vi "Reports.vi"(8 "Reports":T1(array[cluster]), 9 "Path In":path) -> ()   [LabVIEW 2018]
panel:
  out "Failed":bool
  out "Numeric 2":dbl
  out "String":string="C:\\LabVIEW_Data\\Default.txt"
  out "Numeric":dbl
  out "Output":string
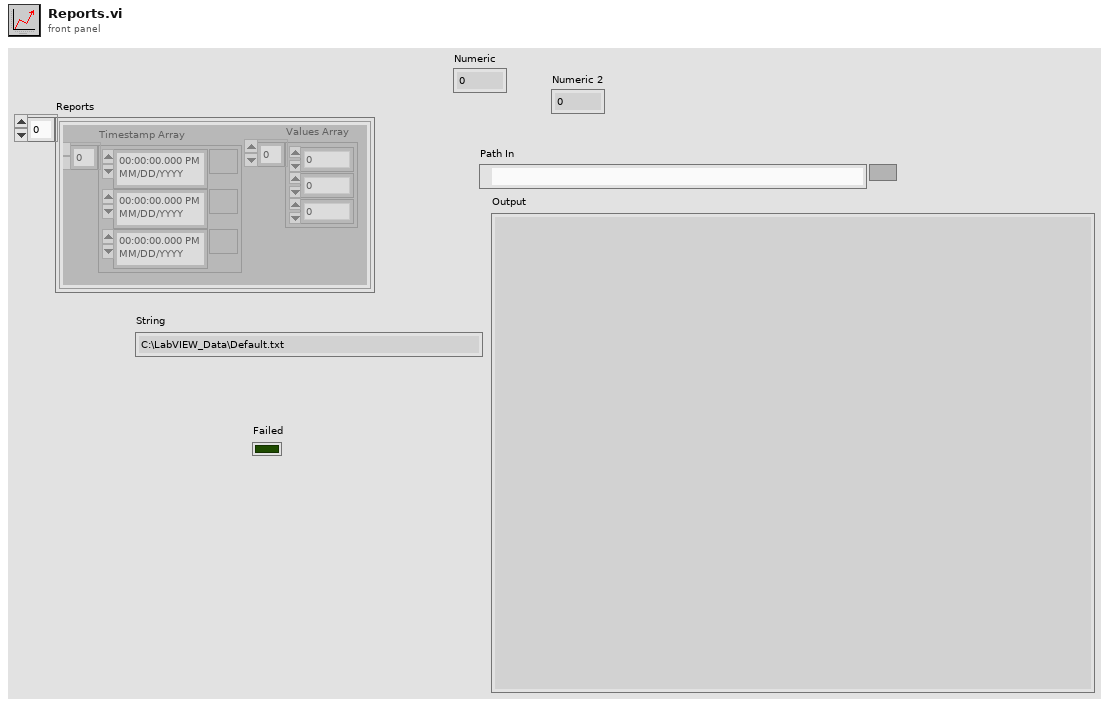
[diagram p1: front panel]
types:
  T1 = cluster{"Values Array":dbl[], "Timestamp Array":timestamp[]}[]
  T2 = cluster{"Values Array":dbl[], "Timestamp Array":timestamp[]}
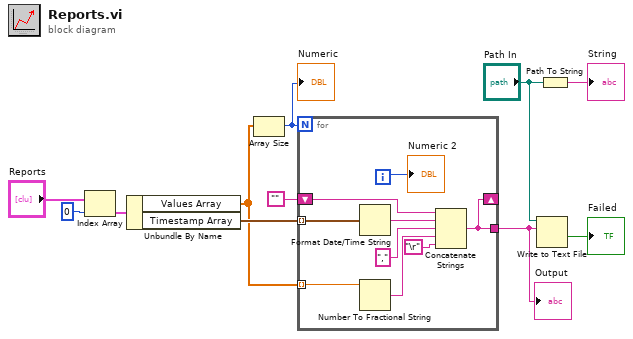
[diagram p0: block diagram]
diagram:
  n1 = Index Array(array="Reports", index=0) -> (element=w9:T2)
  n2 = Unbundle By Name(w9) -> ("Values Array"=w6:dbl[], "Timestamp Array"=w8:timestamp[])
  n3 = Array Size(array=w6) -> (size(s)=w2:i32)
  "Numeric" <- w2
  n4 = for {
    N: w2 -> [_]
    tunnel: w8 -> [w19] mode=indexing
    tunnel: w6 -> [w15] mode=indexing
    shift-right: [w13] -> _
    shift-left: "" -> [w14]
    tunnel: [w13] -> w7
    i -> [w12]
    n5 = Format Date/Time String(seconds (now)=w19) -> (date/time string=w18:string)  [unwired: 2 in]
    n6 = Number To Fractional String(number=w15) -> (F-format string=w16:string)  [unwired: 3 in]
    n7 = Concatenate Strings(w14, w18, ",", w16, "\r") -> (w13:string)
    "Numeric 2" <- w12
  }
  "Output" <- w7
  n8 = Write to Text File(file (use dialog)="Path In", text=w7) -> (cancelled=→"Failed":bool)  [unwired: 2 in, 2 out]
  n9 = Path To String(path="Path In") -> (string=→"String":string)
